vi "Parse ERD Write Expected Data (Rev 2 API).vi"(0 "ERD Write Data In":T1 {"ERD Number" format="%.0x"}, 5 "Request ID":string, 11 "Error In":errorcluster) -> (8 "Expected Data":string, 15 "Error Out":errorcluster)   [LabVIEW 2023, in "GEA2_Toolkit.lvlib"]
uses:
  library/GEA2_Toolkit.lvlib
  type defs/ERD Write Data In.ctl
  type defs/Data Type.ctl
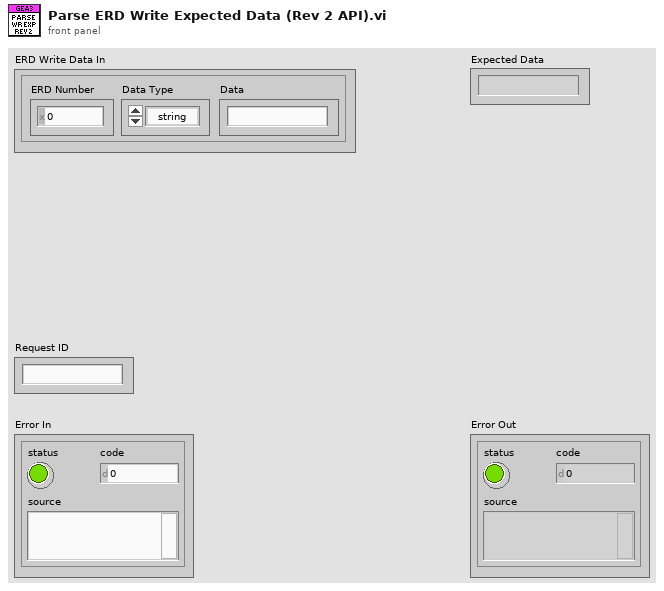
[diagram p1: front panel]
types:
  T1 = typedef "ERD Write Data In.ctl" = cluster{"ERD Number":u16, "Data Type":T2, "Data":string}
  T2 = typedef "Data Type.ctl" = enum16{"string", "boolean", "uint8_t", "uint16_t", "uint32_t", "uint64_t", "int8_t", "int16_t", "int32_t", "int64_t"}
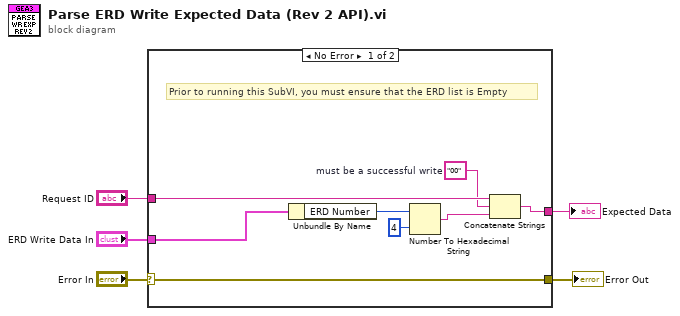
[diagram p0: block diagram]
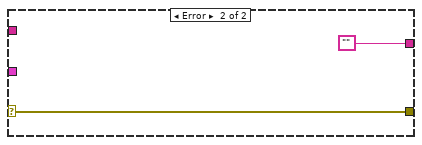
[diagram p2: hidden frame]
diagram:
  n1 = case shown="No Error" "Error In" {
    selector: "Error In" -> [w11 w15]
    tunnel: [w12 ""] -> w5
    tunnel: "ERD Write Data In" -> [w6 _]
    tunnel: [w11 w15] -> w3
    tunnel: "Request ID" -> [w8 _]
    frame No Error {
      w7 = "00"  # must be a successful write
      # "Prior to running this SubVI, you must ensure that the ERD list is Empty"
      n2 = Unbundle By Name(w6) -> ("ERD Number"=w10:u16)
      n3 = Number To Hexadecimal String(1:i16 4 ("width (-)"), 2:w10) -> (0:w13:string)
      n4 = Concatenate Strings(w8, w7, w13) -> (w12:string)
    }
    frame Error {
    }
  }
  "Expected Data" <- w5
  "Error Out" <- w3
